vi "create file paths.vi"(8 "error in":errorcluster) -> (0 "error out":errorcluster, 3 "File path":T1={"configuration"=path "c:/Parametros.cfg", "confRFID"=path "c:/RFID/TAGS.csv", "LOG.txt"=path "", "Path LOG"=path "c:/TEST", "Path_data"=path "c:/Trenes", "TAGS leidos"=path "c:/RFID/TAGS.csv", "configuracion flota"=path "", "flota"=path "", "Nombre de archivo"=[], "Folder calibration"=path "", "calibration log"=path "", "Reporting Procesamiento"=path "", "Error ejes"=path "", "Reporting Adquisición"=path ""})   [LabVIEW 2015]
uses:
  controls/File paths.ctl
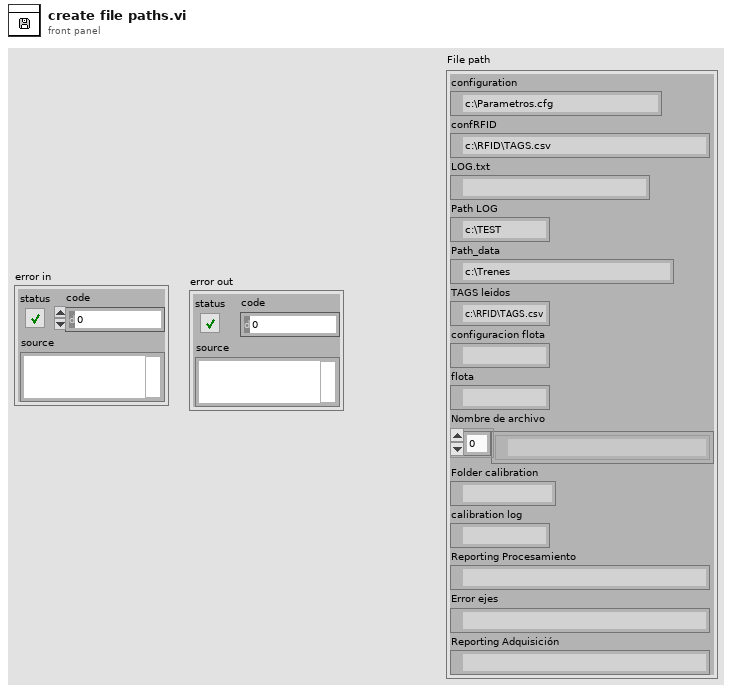
[diagram p1: front panel]
types:
  T1 = typedef "File paths.ctl" = cluster{"configuration":path, "confRFID":path, "LOG.txt":path, "Path LOG":path, "Path_data":path, "TAGS leidos":path, "configuracion flota":path, "flota":path, "Nombre de archivo":path[], "Folder calibration":path, "calibration log":path, "Reporting Procesamiento":path, "Error ejes":path, "Reporting Adquisición":path}
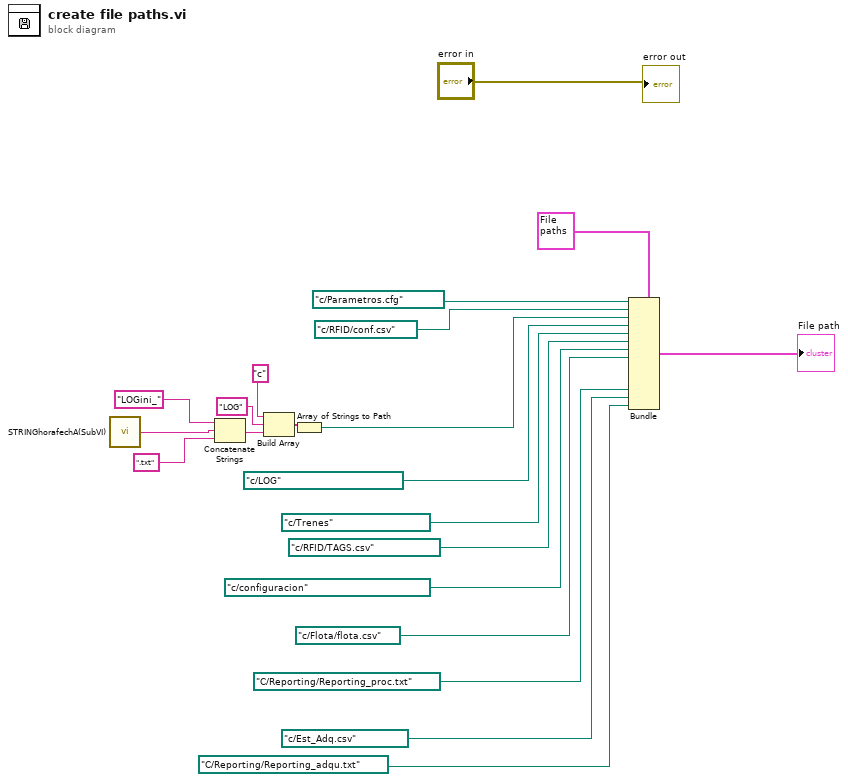
[diagram p0: block diagram]
diagram:
  n1 = call "STRINGhorafechA(SubVI).vi"() -> ("STRINGhora_fecha"=w16:string)
  n2 = Concatenate Strings("LOGini_" ("string"), w16, ".txt" ("string")) -> (w18:string)
  n3 = Build Array("c", "LOG" ("element"), w18) -> (w15:string[])
  n4 = Array of Strings to Path(0:w15) -> (2:w11:path)  [unwired: 1 out]
  n5 = Bundle(cluster=T1 {"configuration"=path "c:/Parametros.cfg", "confRFID"=path "c:/RFID/TAGS.csv", "LOG.txt"=path "", "Path LOG"=path "c:/TEST", "Path_data"=path "c:/Trenes", "TAGS leidos"=path "c:/RFID/TAGS.csv", "configuracion flota"=path "", "flota"=path "", "Nombre de archivo"=[], "Folder calibration"=path "", "calibration log"=path "", "Reporting Procesamiento"=path "", "Error ejes"=path "", "Reporting Adquisición"=path ""} ("File path"), "configuration"=path "c:/Parametros.cfg" ("configuration file path"), "confRFID"=path "c:/RFID/conf.csv" ("file path (use dialog)"), "LOG.txt"=w11, "Path LOG"=path "c:/LOG" ("file path (use dialog)"), "Path_data"=path "c:/Trenes" ("file path (use dialog)"), "TAGS leidos"=path "c:/RFID/TAGS.csv" ("file path (use dialog)"), "configuracion flota"=path "c:/configuracion" ("file path (dialog if empty)"), "flota"=path "c:/Flota/flota.csv" ("Path"), "Reporting Procesamiento"=path "C:/Reporting/Reporting_proc.txt" ("file (use dialog)"), "Error ejes"=path "c:/Est_Adq.csv" ("file path (use dialog)"), "Reporting Adquisición"=path "C:/Reporting/Reporting_adqu.txt" ("file (use dialog)")) -> (→"File path":T1)  [unwired: 3 in]
  "error out" <- "error in"
